vi "MGCC_MdlMgmt_RTDS_dynamic.vi"() -> ()   [LabVIEW 2016]
uses:
  <vilib>/imath/engines/lvmath2/RunTimeEngine/IndexRead/NIMS M($,S).vi
  <vilib>/imath/engines/lvmath2/RunTimeEngine/BuiltInFunctions/length/NIMS_length(GV).vi
  <vilib>/imath/engines/lvmath2/RunTimeEngine/BuiltInFunctions/zeros/NIMS_M=zeros(I32,I32).vi
  <vilib>/imath/engines/lvmath2/RunTimeEngine/ErrorHandling/NIMS_Create Error From Enums.vi
  <vilib>/imathl/engines/lvmath/Functions/Error Handling/Create Error.vi
  <vilib>/imath/engines/lvmath2/RunTimeEngine/IndexReplace/NIMS M(S,$)=V.vi
  <vilib>/imath/engines/lvmath2/RunTimeEngine/RangeToken/NIMS_Range_R3 - Integer.vi
  <vilib>/imath/engines/lvmath2/RunTimeEngine/IndexRead/NIMS M(S,S).vi
  <vilib>/imath/engines/lvmath2/RunTimeEngine/IndexRead/NIMS M(S,R2).vi
  <vilib>/imath/engines/lvmath2/RunTimeEngine/BuiltInFunctions/is_membermx/NIMS_is_membermx(GM,GM).vi
  <vilib>/imath/engines/lvmath2/RunTimeEngine/BuiltInFunctions/sum/NIMS_sum(GM,Sca).vi
  <vilib>/imath/engines/lvmath2/RunTimeEngine/IndexReplace/NIMS M(S,S)=S.vi
  <vilib>/imath/engines/lvmath2/RunTimeEngine/BuiltInFunctions/sum/NIMS_sum(GV).vi
  <vilib>/imath/engines/lvmath2/RunTimeEngine/BuiltInFunctions/findnz/NIMS_[1o]_findnz(GRowV).vi
  <vilib>/imath/engines/lvmath2/RunTimeEngine/IndexRead/NIMS M($,V).vi
  <vilib>/imath/engines/lvmath2/RunTimeEngine/BuiltInFunctions/sets_union/NIMS_sets_union(GV2).vi
  <vilib>/imath/engines/lvmath2/RunTimeSupport/NIMS_Get Any Vector_w Error - Matrix.vi
  <vilib>/imath/engines/lvmath2/RunTimeEngine/BuiltInFunctions/zeros/NIMS_V=zeros(I32,I32).vi
  <vilib>/imath/engines/lvmath2/RunTimeEngine/IndexReplace/NIMS M($,V)=V.vi
  <vilib>/imath/engines/lvmath2/RunTimeEngine/RangeToken/NIMS_Range.vi
  <vilib>/imath/engines/lvmath2/RunTimeEngine/CommandStatement/MC_CommandStatement_break.vi
  <vilib>/imath/engines/lvmath2/RunTimeEngine/BuiltInFunctions/is_membermx/NIMS_is_membermx(GV,GM).vi
  <vilib>/imath/engines/lvmath2/RunTimeEngine/IndexRead/NIMS V(S).vi
  <vilib>/imath/engines/lvmath2/RunTimeSupport/NIMS_Error if Not Equal.vi
  <vilib>/imath/engines/lvmath2/RunTimeEngine/BuiltInFunctions/findnz/NIMS_[1o]_findnz(GColV).vi
  <vilib>/imath/engines/lvmath2/RunTimeEngine/IndexRead/NIMS V(V).vi
  <vilib>/imath/engines/lvmath2/RunTimeEngine/IndexReplace/NIMS M(S,S)=V.vi
  <vilib>/imath/engines/lvmath2/RunTimeEngine/IndexRead/NIMS M(M).vi
  <vilib>/imath/engines/lvmath2/RunTimeEngine/IndexReplace/NIMS M(S,S)=M.vi
  <vilib>/imath/engines/lvmath2/RunTimeEngine/IndexReplace/NIMS V(V)=V.vi
  <vilib>/imath/engines/lvmath2/RunTimeEngine/IndexReplace/NIMS M(V,V)=S.vi
  <vilib>/imath/engines/lvmath2/RunTimeEngine/IndexReplace/NIMS M(V,V)=V.vi
  <vilib>/imath/engines/lvmath2/RunTimeEngine/NodeEndStatement/NIMS_NodeEndStatement_Output.vi
  <vilib>/imath/engines/lvmath2/RunTimeEngine/ErrorHandling/NIMS_Finalize Error.vi
panel:
  out "Array":dbl[][][](array[numeric])
  in  "Node switch status 8":bool
  in  "Node switch status 7":bool
  in  "Node switch status 6":bool
  in  "Node switch status 5":bool
  in  "Node switch status 4":bool
  in  "Node switch status 3":bool
  in  "Node switch status 2":bool
  in  "Node switch status 1":bool
  out "f_MGCC_MdlMgmt_Topology_RTDS 2":dbl[][](array[numeric])
  out "B1":dbl[][](array[numeric])
  out "B 2":dbl[][](array[numeric])
  out "f_MGCC_MdlMgmt_Topology_RTDS":dbl[][](array[numeric])
  out "C":dbl[][](array[numeric])
  out "error out":errorcluster
  out "S4":bool
  out "S3":bool
  out "S2":bool
  out "S1":bool
  out "PV":bool
  out "G2":bool
  out "G1":bool
  out "B":bool
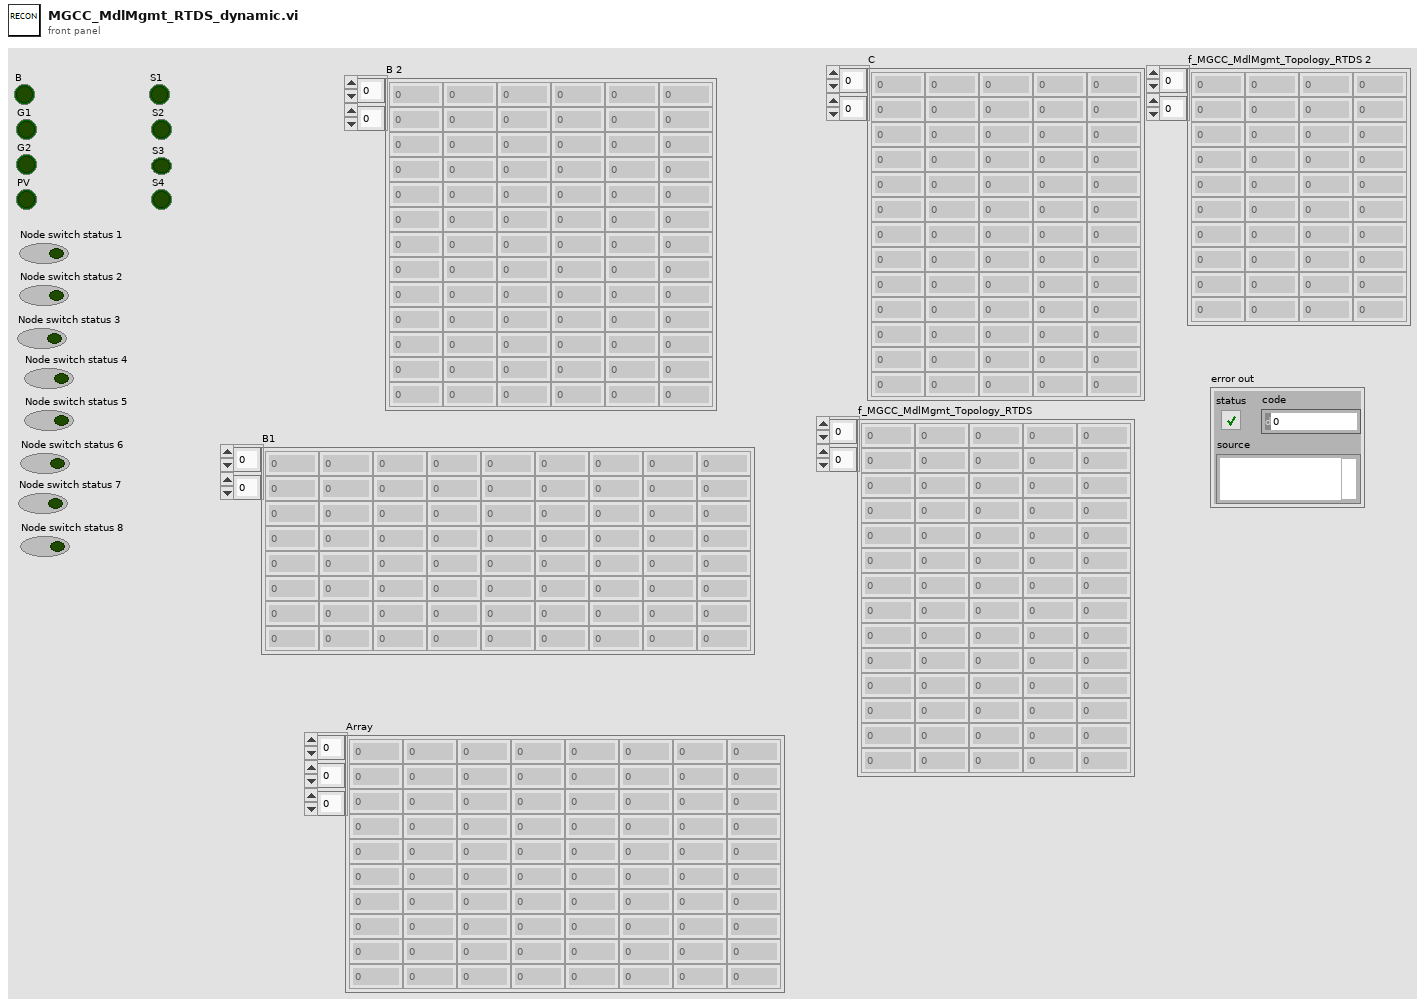
[diagram p1: front panel]
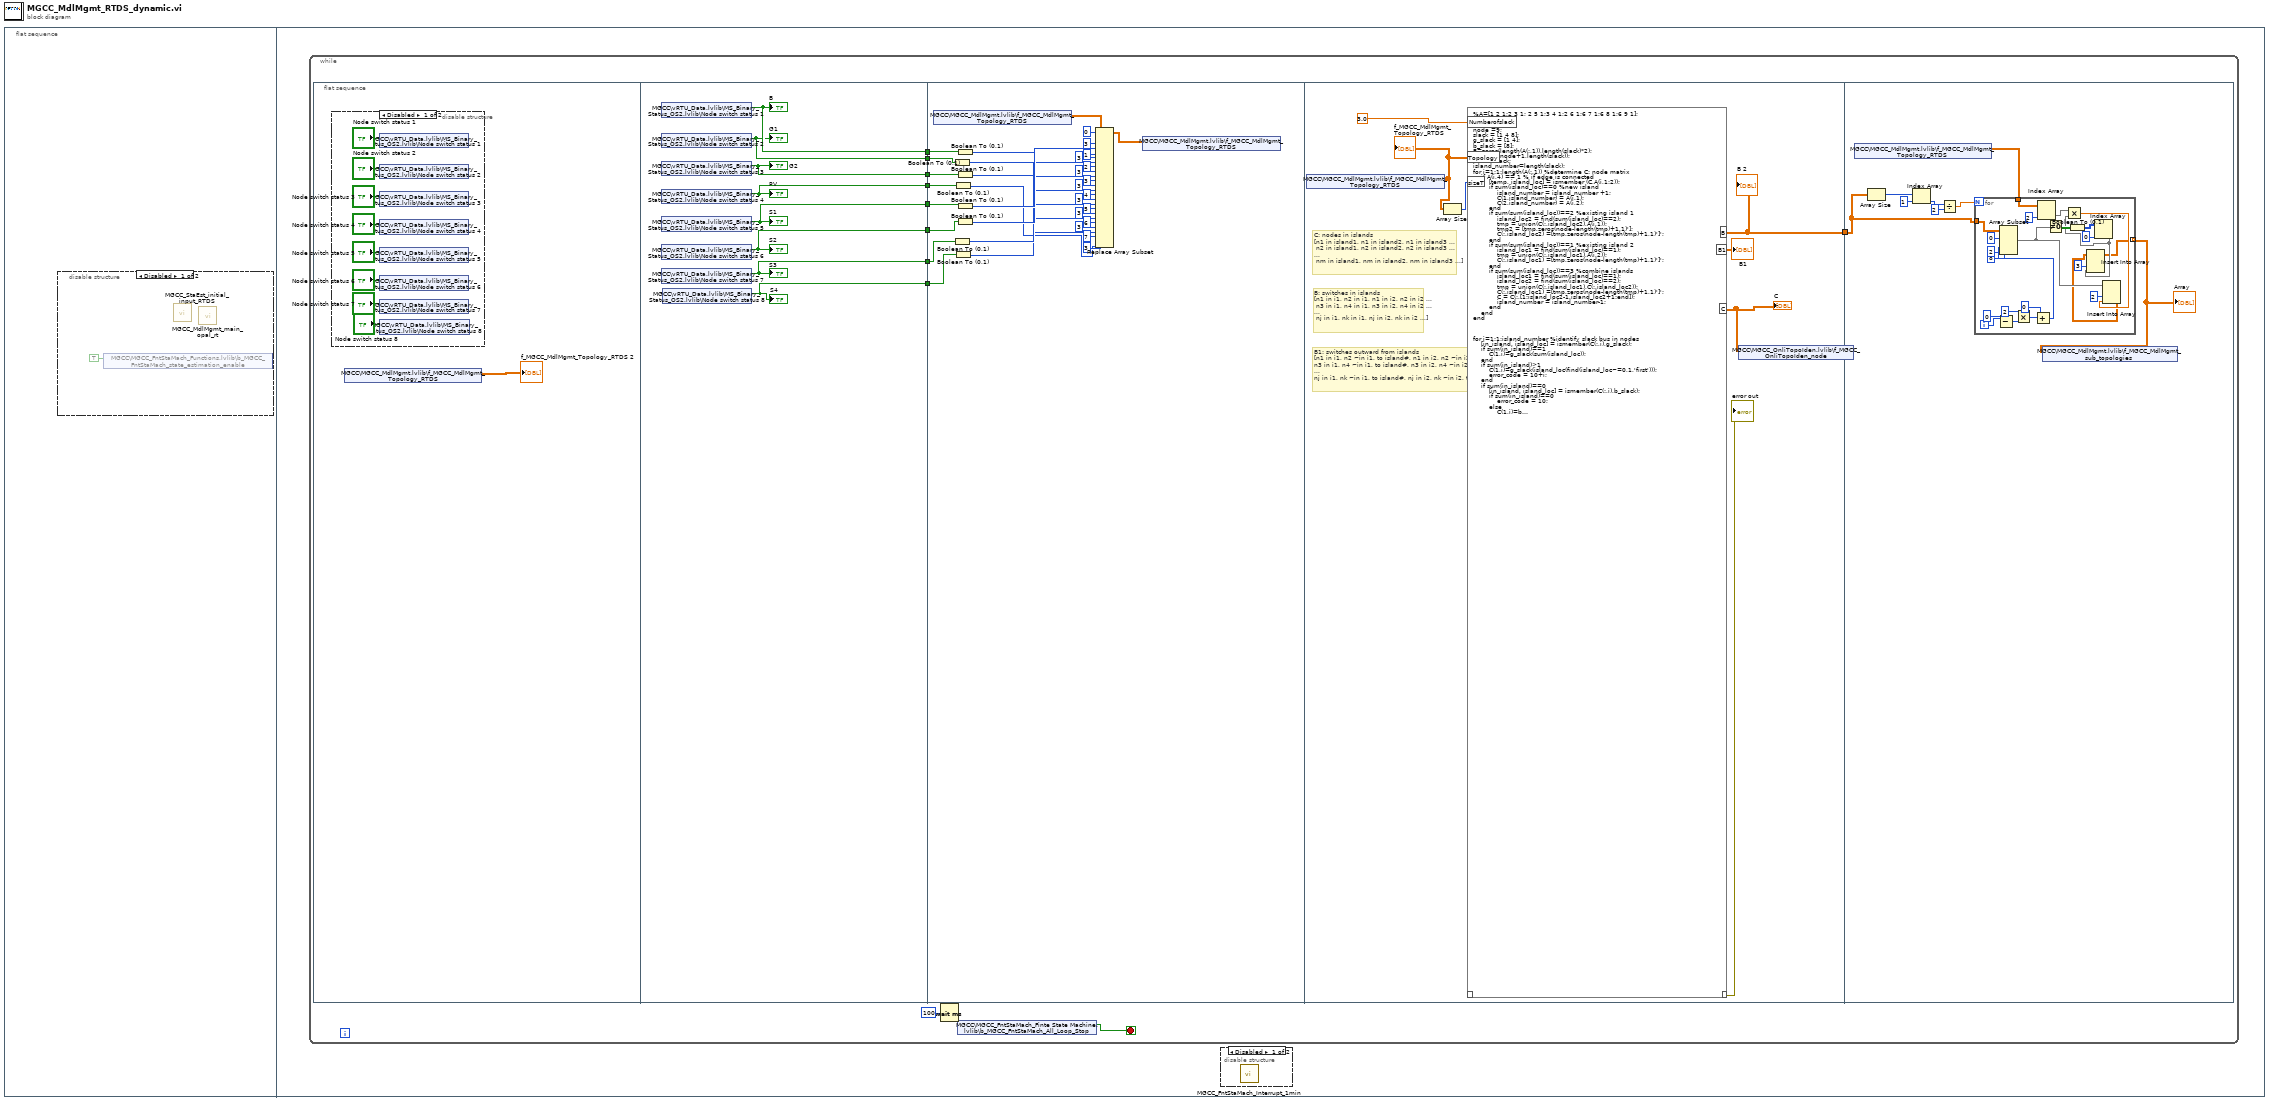
[diagram p0: block diagram]
diagram:
  n1 = flat-sequence {
    frame #0 {
      n2 = disable-structure shown="Disabled" {
        frame Disabled {
          n3 = shared-variable "MGCC\\MGCC_FntStaMach_Functions.lvlib\\b_MGCC_FntStaMach_state_estimation_enable"(TRUE ("b_MGCC_FntStaMach_state_estimation_enable")) -> ()  [unwired: 1 in, 1 out]
          n4 = call "MGCC_StaEst_initial_input_RTDS.vi"() -> ()  [unwired: 11 in, 1 out]
          n5 = call "MGCC_MdlMgmt_main_opal_rt.vi"() -> ()  [unwired: 12 in]
        }
        frame Enabled {
        }
      }
    }
    frame #1 {
      n6 = while {
        stop <- w2 stop-if-true
        n7 = flat-sequence {
          tunnel: [w29] -> w12
          tunnel: [w28] -> w11
          tunnel: [w27] -> w10
          tunnel: [w26] -> w9
          tunnel: [w25] -> w8
          tunnel: [w24] -> w7
          tunnel: [w23] -> w6
          tunnel: [w22] -> w5
          tunnel: w12 -> [w61]
          tunnel: w11 -> [w60]
          tunnel: w10 -> [w59]
          tunnel: w9 -> [w58]
          tunnel: w8 -> [w38]
          tunnel: w7 -> [w37]
          tunnel: w6 -> [w36]
          tunnel: w5 -> [w35]
          tunnel: [w67] -> w3
          tunnel: w3 -> [w2105]
          frame #0 {
            n8 = disable-structure shown="Disabled" {
              frame Disabled {
                n9 = shared-variable "MGCC\\vRTU_Data.lvlib\\MS_Binary_Status_OS2.lvlib\\Node switch status 1"("Node switch status 1") -> ()  [unwired: 1 in, 1 out]
                n10 = shared-variable "MGCC\\vRTU_Data.lvlib\\MS_Binary_Status_OS2.lvlib\\Node switch status 2"("Node switch status 2") -> ()  [unwired: 1 in, 1 out]
                n11 = shared-variable "MGCC\\vRTU_Data.lvlib\\MS_Binary_Status_OS2.lvlib\\Node switch status 3"("Node switch status 3") -> ()  [unwired: 1 in, 1 out]
                n12 = shared-variable "MGCC\\vRTU_Data.lvlib\\MS_Binary_Status_OS2.lvlib\\Node switch status 4"("Node switch status 4") -> ()  [unwired: 1 in, 1 out]
                n13 = shared-variable "MGCC\\vRTU_Data.lvlib\\MS_Binary_Status_OS2.lvlib\\Node switch status 5"("Node switch status 5") -> ()  [unwired: 1 in, 1 out]
                n14 = shared-variable "MGCC\\vRTU_Data.lvlib\\MS_Binary_Status_OS2.lvlib\\Node switch status 6"("Node switch status 6") -> ()  [unwired: 1 in, 1 out]
                n15 = shared-variable "MGCC\\vRTU_Data.lvlib\\MS_Binary_Status_OS2.lvlib\\Node switch status 7"("Node switch status 7") -> ()  [unwired: 1 in, 1 out]
                n16 = shared-variable "MGCC\\vRTU_Data.lvlib\\MS_Binary_Status_OS2.lvlib\\Node switch status 8"("Node switch status 8") -> ()  [unwired: 1 in, 1 out]
              }
              frame Enabled {
              }
            }
            n17 = shared-variable "MGCC\\MGCC_MdlMgmt.lvlib\\f_MGCC_MdlMgmt_Topology_RTDS"() -> (→"f_MGCC_MdlMgmt_Topology_RTDS 2":dbl[][])  [unwired: 1 in, 1 out]
          }
          frame #1 {
            n18 = shared-variable "MGCC\\vRTU_Data.lvlib\\MS_Binary_Status_OS2.lvlib\\Node switch status 1"() -> (w25:bool)  [unwired: 1 in, 1 out]
            "B" <- w25
            n19 = shared-variable "MGCC\\vRTU_Data.lvlib\\MS_Binary_Status_OS2.lvlib\\Node switch status 2"() -> (w24:bool)  [unwired: 1 in, 1 out]
            "G1" <- w24
            n20 = shared-variable "MGCC\\vRTU_Data.lvlib\\MS_Binary_Status_OS2.lvlib\\Node switch status 3"() -> (w23:bool)  [unwired: 1 in, 1 out]
            "G2" <- w23
            n21 = shared-variable "MGCC\\vRTU_Data.lvlib\\MS_Binary_Status_OS2.lvlib\\Node switch status 4"() -> (w22:bool)  [unwired: 1 in, 1 out]
            "PV" <- w22
            n22 = shared-variable "MGCC\\vRTU_Data.lvlib\\MS_Binary_Status_OS2.lvlib\\Node switch status 5"() -> (w29:bool)  [unwired: 1 in, 1 out]
            "S1" <- w29
            n23 = shared-variable "MGCC\\vRTU_Data.lvlib\\MS_Binary_Status_OS2.lvlib\\Node switch status 6"() -> (w28:bool)  [unwired: 1 in, 1 out]
            "S2" <- w28
            n24 = shared-variable "MGCC\\vRTU_Data.lvlib\\MS_Binary_Status_OS2.lvlib\\Node switch status 7"() -> (w27:bool)  [unwired: 1 in, 1 out]
            "S3" <- w27
            n25 = shared-variable "MGCC\\vRTU_Data.lvlib\\MS_Binary_Status_OS2.lvlib\\Node switch status 8"() -> (w26:bool)  [unwired: 1 in, 1 out]
            "S4" <- w26
          }
          frame #2 {
            n26 = shared-variable "MGCC\\MGCC_MdlMgmt.lvlib\\f_MGCC_MdlMgmt_Topology_RTDS"() -> (w63:dbl[][])  [unwired: 1 in, 1 out]
            n27 = Boolean To (0,1)(Boolean=w37) -> (0, 1=w33:i16)
            n28 = Boolean To (0,1)(Boolean=w59) -> (0, 1=w40:i16)
            n29 = Boolean To (0,1)(Boolean=w35) -> (0, 1=w31:i16)
            n30 = Boolean To (0,1)(Boolean=w58) -> (0, 1=w39:i16)
            n31 = Boolean To (0,1)(Boolean=w38) -> (0, 1=w34:i16)
            n32 = Boolean To (0,1)(Boolean=w36) -> (0, 1=w32:i16)
            n33 = Boolean To (0,1)(Boolean=w61) -> (0, 1=w42:i16)
            n34 = Boolean To (0,1)(Boolean=w60) -> (0, 1=w41:i16)
            n35 = Replace Array Subset(array=w63, new element #1=w42, index (row) #1=0 ("disabled index (row)"), index (col) #1=3 ("disabled index (col)"), new element #2=w41, index (row) #2=1 ("index (row)"), index (col) #2=3 ("disabled index (col)"), new element #3=w40, index (row) #3=2 ("index (row)"), index (col) #3=3 ("disabled index (col)"), new element #4=w39, index (row) #4=3 ("index (row)"), index (col) #4=3 ("disabled index (col)"), new element #5=w33, index (row) #5=4 ("index (row)"), index (col) #5=3 ("disabled index (col)"), new element #6=w32, index (row) #6=5 ("index (row)"), index (col) #6=3 ("disabled index (col)"), new element #7=w34, index (row) #7=6 ("index (row)"), index (col) #7=3 ("disabled index (col)"), new element #8=w31, index (row) #8=7 ("index (row)"), index (col) #8=3 ("disabled index (col)")) -> (w30:dbl[][])
            n36 = shared-variable "MGCC\\MGCC_MdlMgmt.lvlib\\f_MGCC_MdlMgmt_Topology_RTDS"(w30) -> ()  [unwired: 1 in, 1 out]
          }
          frame #3 {
            # "B1: switches outward from islands\n[n1 in i1, n2 ~in i1, to island#, n1 in i2, n2 ~in i2, to island#, ...\nn3 in i1, n4 ~in i1, to island#, n3 in i2, n4 ~in i2, to island#, ...\n...\nnj in i1, nk ~in i1, to island#, nj in i2, nk ~in i2, to island#, ...]"
            # "B: switches in islands\n[n1 in i1, n2 in i1, n1 in i2, n2 in i2 ...\n n3 in i1, n4 in i1, n3 in i2, n4 in i2 ...\n...\n nj in i1, nk in i1, nj in i2, nk in i2 ...]"
            # "C: nodes in islands\n[n1 in island1, n1 in island2, n1 in island3 ...\n n2 in island1, n2 in island2, n2 in island3 ...\n...\n nm in island1, nm in island2, nm in island3 ...]"
            n37 = shared-variable "MGCC\\MGCC_MdlMgmt.lvlib\\f_MGCC_MdlMgmt_Topology_RTDS"() -> (w69:dbl[][])  [unwired: 1 in, 1 out]
            "f_MGCC_MdlMgmt_Topology_RTDS" <- w69
            n38 = Array Size(array=w69) -> (size(s)=w68:i32[])
            n39 = mathscript code="%A=[1 2 1;2 3 1; 2 5 1;3 4 1;2 6 1;6 7 1;6 8 1;6 9 1];\nA=Topology;\ni=0; j=0;\nnode =9;\nslack = [1 4 8];\ng_slack = [1 4];\nb_slack = [8];\nB=zeros(length(A(:,1)),length(slack)*2);\nC=zeros(node+1,length(slack));\nC(2,:)=slack;\nisland_number=length(slack);\nfor i=1:1:length(A(:,1)) %determine C: node matrix\n    if A(i,4) == 1 % if edge is connected\n        [temp, island_loc] = ismember (C,A(i,1:2));\n        if sum(island_loc)==0 %new island\n            island_number = island_number +1;\n            C(1,island_number) = A(i,1);\n            C(2,island_number) = A(i,2);\n        end\n        if sum(sum(island_loc))==2 %existing island 1\n            island_loc2 = find(sum(island_loc)==2);\n            tmp = union(C(:,island_loc2),A(i,1));\n            tmp2 = [tmp,zeros(node-length(tmp)+1,1)'];\n            C(:,island_loc2) =[tmp,zeros(node-length(tmp)+1,1)']';\n        end\n        if sum(sum(island_loc))==1 %existing island 2\n            island_loc1 = find(sum(island_loc)==1);\n            tmp = union(C(:,island_loc1),A(i,2));\n            C(:,island_loc1) =[tmp,zeros(node-length(tmp)+1,1)']';\n        end\n        if sum(sum(island_loc))==3 %combine islands\n            island_loc1 = find(sum(island_loc)==1);\n            island_loc2 = find(sum(island_loc)==2);\n            tmp = union(C(:,island_loc1),C(:,island_loc2));\n            C(:,island_loc1) =[tmp,zeros(node-length(tmp)+1,1)']';\n            C = C(:,[1:island_loc2-1,island_loc2+1:end]);\n            island_number = island_number-1;\n        end\n    end\nend\n\n\n\nfor i=1:1:island_number %identify slack bus in nodes\n    [in_island, island_loc] = ismember(C(:,i),g_slack);\n    if sum(in_island)==1\n        C(1,i)=g_slack(sum(island_loc));\n    end\n    if sum(in_island)>1\n        C(1,i)=g_slack(island_loc(find(island_loc~=0,1,'first')));\n        error_code = 10+i;\n    end\n    if sum(in_island)==0\n        [in_island, island_loc] = ismember(C(:,i),b_slack);\n        if sum(in_island)==0\n            error_code = 10;\n        else\n            C(1,i)=b_slack(island_loc(find(island_loc~=0,1,'first')));\n        end\n    end\nend\n\nB_index = zeros(1,island_number);\nB = zeros(1,island_number*2);\nB1_index = zeros(1,island_number);\nB1 = zeros(1,island_number*3);\nfor i=1:1:length(A(:,1))\n    if A(i,4) == 1 % if edge is connected\n        [in_island, island_loc] = ismember (C,A(i,1));\n        island_loc1 = find(sum(island_loc)~=0,1,'first');\n        B_index(island_loc1) = B_index(island_loc1)+1;\n        \n        B(B_index(island_loc1),island_loc1*2-1) = A(i,1);\n        B(B_index(island_loc1),island_loc1*2) = A(i,2);\n    end\n    if A(i,4) ==0 %if edge is not connected\n        island_loc1 = 0; island_loc2 = 0;\n        [in_island, island_loc] = ismember (C,A(i,1));\n        island_loc1 = find(sum(island_loc)~=0,1,'first');\n        [in_island, island_loc] = ismember (C,A(i,2));\n        island_loc2 = find(sum(island_loc)~=0,1,'first');\n        if island_loc1>0\n            B1_index(island_loc1) = B1_index(island_loc1) +1;\n            B1(B1_index(island_loc1),island_loc1*3-2) = A(i,1);\n            B1(B1_index(island_loc1),island_loc1*3-1) = A(i,2);\n            if island_loc2 > 0\n                B1(B1_index(island_loc1),island_loc1*3) = island_loc2;\n            else\n                B1(B1_index(island_loc1),island_loc1*3) = 0;\n            end\n        end\n        if island_loc2>0 %right terminal in island, non-critical line\n            B1_index(island_loc2) = B1_index(island_loc2) +1;\n            B1(B1_index(island_loc2),island_loc2*3-2) = A(i,2);\n            B1(B1_index(island_loc2),island_loc2*3-1) = A(i,1);\n            if island_loc1 > 0\n                B1(B1_index(island_loc2),island_loc2*3) = island_loc1;\n            else\n                B1(B1_index(island_loc2),island_loc2*3) = 0;\n            end\n        end\n    end   \nend"("Numberofslack"=3.0, "Topology"=w69, "sizeT"=w68) -> ("??"=→"error out":errorcluster, "B"=w67:dbl[][], "C"=w64:dbl[][], "B1"=→"B1":dbl[][])  [unwired: 1 in]
            "C" <- w64
            "B 2" <- w67
            n40 = shared-variable "MGCC\\MGCC_OnliTopoIden.lvlib\\f_MGCC_OnliTopoIden_node"(w64) -> ()  [unwired: 1 in, 1 out]
          }
          frame #4 {
            n41 = shared-variable "MGCC\\MGCC_MdlMgmt.lvlib\\f_MGCC_MdlMgmt_Topology_RTDS"() -> (w2103:dbl[][])  [unwired: 1 in, 1 out]
            n42 = Array Size(array=w2105) -> (size(s)=w2110:i32[])
            n43 = Index Array(array=w2110, index=1) -> (element=w2108:i32)
            n44 = Divide(x=w2108, y=2) -> (x/y=w2106:dbl)
            n45 = for {
              N: w2106 -> [_]
              tunnel: w2105 -> [w2134]
              tunnel: [w2111] -> w2104 mode=indexing
              tunnel: w2103 -> [w2119]
              i -> [w2132]
              n46 = Subtract(x=w2132, y=0) -> (x-y=w2130:i32)
              n47 = Multiply(x=2, y=w2130) -> (x*y=w2128:i32)
              n48 = Add(x=w2128, y=0) -> (x+y=w2126:i32)
              n49 = Array Subset(array=w2134, index (row)=0 ("index"), length (row)=8 ("length"), index (col)=w2126, length (col)=2 ("length")) -> (w2113:dbl[][])
              n50 = Index Array(array=w2119, index (col)=2 ("disabled index (col)")) -> (element=w2117:dbl[])  [unwired: 1 in]
              n51 = Not Equal To 0?(x=w2113) -> (x != 0?=w2123:bool[][])
              n52 = Boolean To (0,1)(Boolean=w2123) -> (0, 1=w2122:i16[][])
              n53 = Index Array(array=w2122, index (col)=0 ("disabled index (col)")) -> (element=w2116:i16[])  [unwired: 1 in]
              n54 = Multiply(x=w2117, y=w2116) -> (x*y=w2115:dbl[])
              n55 = Insert Into Array(array=w2113, index (col)=2 ("disabled index (col)"), new element=w2115) -> (w2112:dbl[][])  [unwired: 1 in]
              n56 = Insert Into Array(array=w2112, index (col)=3 ("disabled index (col)"), new element=w2116) -> (w2111:dbl[][])  [unwired: 1 in]
            }
            "Array" <- w2104
            n57 = shared-variable "MGCC\\MGCC_MdlMgmt.lvlib\\f_MGCC_MdlMgmt_sub_topologies"(w2104) -> ()  [unwired: 1 in, 1 out]
          }
        }
        n58 = Wait (ms)(milliseconds to wait=u32 100) -> ()  [unwired: 1 out]
        n59 = shared-variable "MGCC\\MGCC_FntStaMach_Finte State Machine.lvlib\\b_MGCC_FntStaMach_All_Loop_Stop"() -> (w2:bool)  [unwired: 1 in, 1 out]
      }
      n60 = disable-structure shown="Disabled" {
        frame Disabled {
          n61 = call "MGCC_FntStaMach_Interrupt_1min.vi"() -> ()  [unwired: 11 in, 1 out]
        }
        frame Enabled {
        }
      }
    }
  }
